vi "3_FM demodulation.vi"() -> ()   [LabVIEW 2022 SP3]
uses:
  <instrlib>/niUSRP/niUSRP Fetch Rx Data (CDB WDT).vi
  <vilib>/measure/maspectr.llb/FFT Power Spectrum and PSD for 1 Chan (CDB).vi
  <vilib>/measure/NI_MAPro.lvlib
  <vilib>/Analysis/NI_AALPro.lvlib
panel:
  out "IQ Plot":waveform(dbl)[](graph)
  in  "Stop Button":bool
  out "Frequency Plot":cluster{"f0":dbl, "df":dbl, "magnitude":dbl[]}(graph)
  in  "device names":refnum<k15>="192.168.10.2"
  in  "active antenna":string="RX1"
  in  "number of samples":i64=10000
  out "error out":errorcluster
  out "coerced gain":dbl=10.0 format="%#_6f"
  out "coerced carrier frequency":dbl=315000000.0 format="%#_6p"
  out "coerced IQ rate":dbl=5000000.0 format="%#_6p"
  in  "gain":dbl=10.0 format="%#_6f"
  in  "carrier frequency":dbl=315000000.0 format="%#_6p"
  in  "IQ rate":dbl=1000000.0 format="%#_6p"
  # "IQ Receiver"
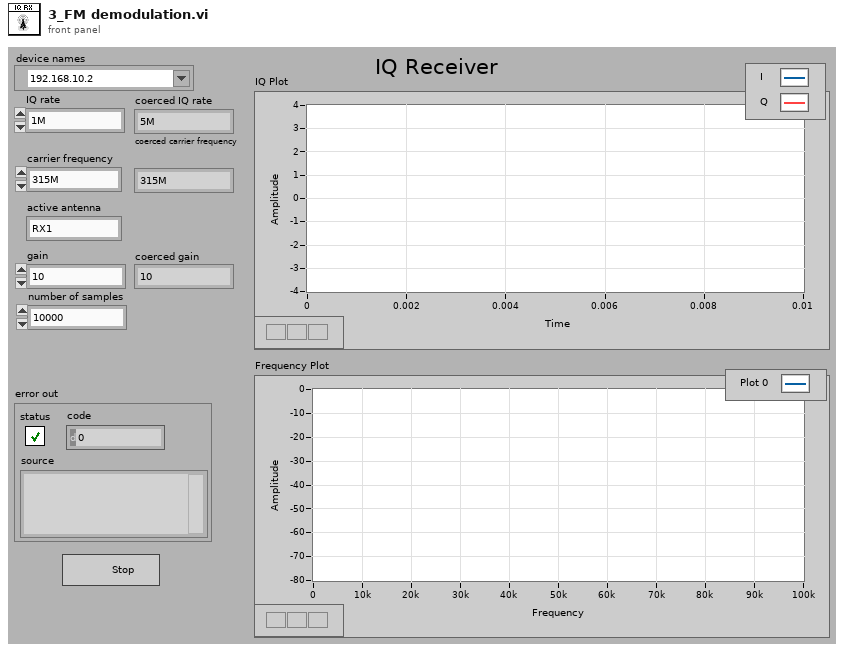
[diagram p1: front panel]
types:
  T1 = typedef "Sound Output Task ID.ctl" = u32
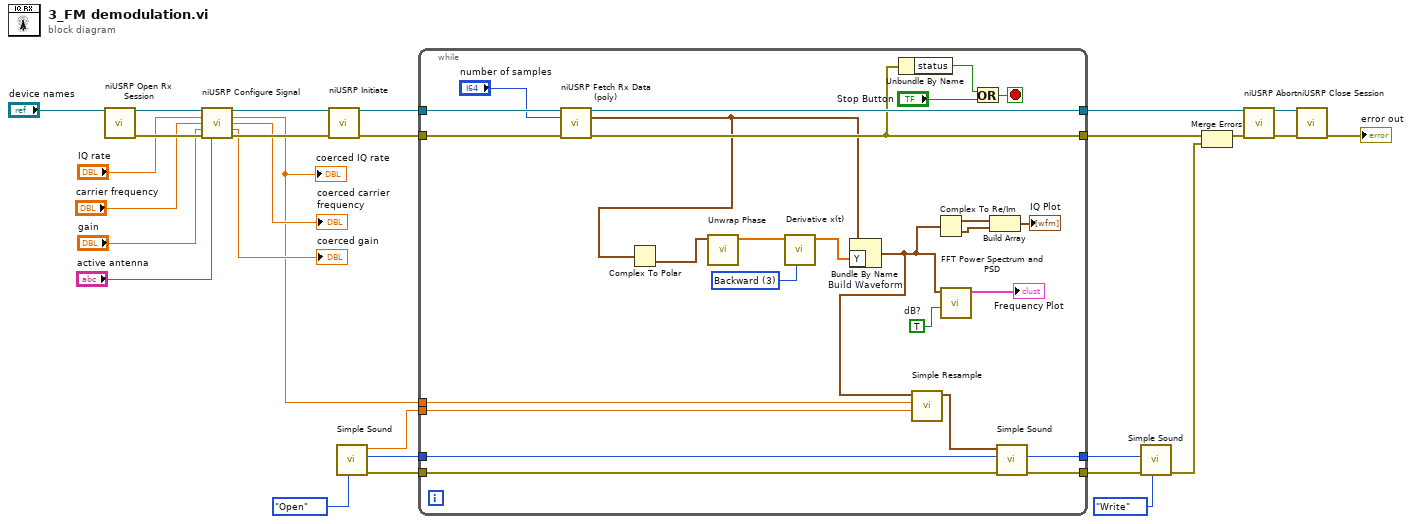
[diagram p0: block diagram]
diagram:
  n1 = call <instrlib>:"niUSRP Open Rx Session.vi"("device names"="device names") -> ("session handle out"=w27:refnum<k15>, "error out"=w26:errorcluster)  [unwired: 13 in]
  n2 = call <instrlib>:"niUSRP Configure Signal.vi"("session handle"=w27, "IQ rate"="IQ rate", "carrier frequency"="carrier frequency", "gain"="gain", "error in (no error)"=w26, "active antenna"="active antenna") -> ("session handle out"=w16:refnum<k15>, "coerced IQ rate"=w5:dbl, "coerced carrier frequency"=→"coerced carrier frequency":dbl, "coerced gain"=→"coerced gain":dbl, "error out"=w18:errorcluster)  [unwired: 5 in]
  "coerced IQ rate" <- w5
  n3 = call <instrlib>:"niUSRP Initiate.vi"("session handle"=w16, "error in (no error)"=w18) -> ("session handle out"=w22:refnum<k15>, "error out"=w21:errorcluster)  [unwired: 12 in]
  n4 = call "Simple Sound.vi"("Action"=enum16{"Open", "Write", "Close"}."Open") -> ("error out"=w3:errorcluster, "task ID out"=w4:T1, "sample rate (S/s)"=w6:dbl)  [unwired: 6 in]
  n5 = while {
    tunnel: w22 -> [w54]
    tunnel: w21 -> [w53]
    tunnel: [w49] -> w12
    tunnel: [w48] -> w10
    tunnel: w6 -> [w44]
    tunnel: w5 -> [w43]
    tunnel: w4 -> [w35]
    tunnel: w3 -> [w34]
    tunnel: [w38] -> w2
    tunnel: [w37] -> w1
    stop <- w47 stop-if-true
    w42 = u16 3 items=["2nd Order Central", "4th Order Central", "Forward", "Backward"] ("method")
    w50 = TRUE  # dB?
    n6 = call-poly <instrlib>:"niUSRP Fetch Rx Data (poly).vi"("session handle"=w54, "number of samples"="number of samples", "error in (no error)"=w53) -> ("session handle out"=w49:refnum<k15>, "data"=w33:waveform(cdb), "error out"=w48:errorcluster)  [unwired: 9 in, 1 out]
    n7 = Complex To Polar(r * e^(i*theta)=w33) -> (theta=w29:waveform(dbl))  [unwired: 1 out]
    n8 = call <vilib>:"Unwrap Phase.vi"("Phase"=w29) -> ("Unwrapped Phase"=w32:dbl[])  [unwired: 9 in, 1 out]
    n9 = call <vilib>:"Derivative x(t).vi"("method"=w42, "X"=w32) -> ("dX/dt"=w31:dbl[])  [unwired: 8 in, 1 out]
    n10 = Bundle By Name "Build Waveform"(cluster=w33, "Y"=w31) -> (w30:waveform(cdb))
    n11 = Unbundle By Name(w48) -> ("status"=w52:bool)
    n12 = call "Simple Resample.vi"("sample rate (S/s)"=w44, "coerced IQ Rate"=w43, "input waveform"=w30) -> ("output waveform"=w36:waveform(dbl))  [unwired: 8 in]
    n13 = Complex To Re/Im(x + iy=w30) -> (x=w41:waveform(dbl), y=w40:waveform(dbl))
    n14 = call-poly <vilib>:"FFT Power Spectrum and PSD.vi"("dB On (F)"=w50, "time signal"=w30) -> ("Power Spectrum / PSD"=→"Frequency Plot":cluster{"f0":dbl, "df":dbl, "magnitude":dbl[]})  [unwired: 6 in, 3 out]
    n15 = Or(x=w52, y="Stop Button") -> (x .or. y?=w47:bool)
    n16 = Build Array(w41, w40) -> (→"IQ Plot":waveform(dbl)[])
    n17 = call "Simple Sound.vi"("error in"=w34, "task ID"=w35, "data"=w36) -> ("error out"=w38:errorcluster, "task ID out"=w37:T1)  [unwired: 4 in, 1 out]
  }
  n18 = call "Simple Sound.vi"("Action"=enum16{"Open", "Write", "Close"}."Write", "error in"=w2, "task ID"=w1) -> ("error out"=w7:errorcluster)  [unwired: 4 in, 2 out]
  n19 = Merge Errors "Merge Errors"(w10, w7) -> (w9:errorcluster)
  n20 = call <instrlib>:"niUSRP Abort.vi"("session handle"=w12, "error in (no error)"=w9) -> ("session handle out"=w24:refnum<k15>, "error out"=w23:errorcluster)  [unwired: 12 in]
  n21 = call <instrlib>:"niUSRP Close Session.vi"("session handle"=w24, "error in (no error)"=w23) -> ("error out"=→"error out":errorcluster)  [unwired: 13 in]
